vi "matlab_create.vi"(4 "error in":errorcluster, 5 "creator":string="h5labview", 6 "platform":string="LabVIEW", 7 "path in":path) -> (0 "error out":errorcluster, 3 "path out":path)   [LabVIEW 2019]
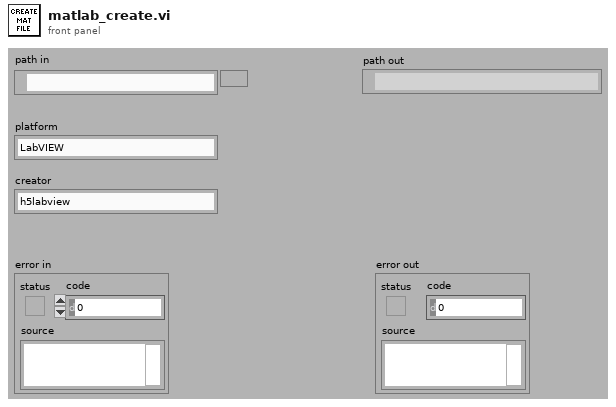
[diagram p1: front panel]
types:
  T1 = enum16{"big-endian, network order", "native, host order", "little-endian"}
  T2 = enum16{"open", "replace", "create", "open or create", "replace or create", "replace or create with confirmation"}
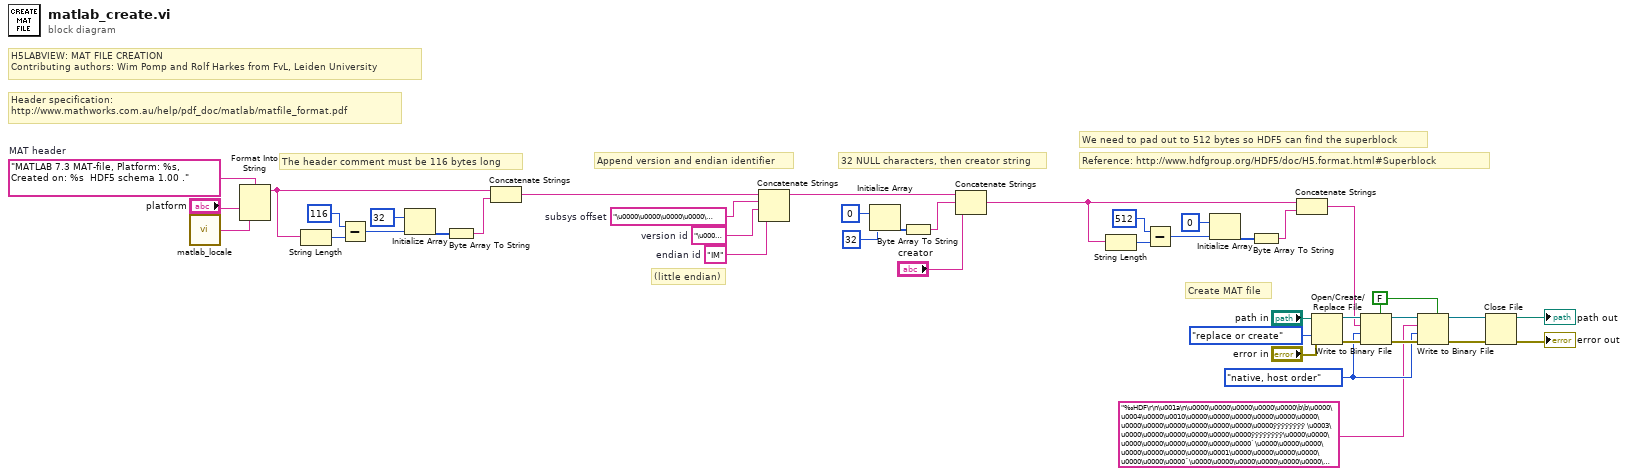
[diagram p0: block diagram]
diagram:
  w4 = T1."native, host order" ("byte order (0:big-endian, network order)")
  w9 = FALSE ("prepend array or string size? (T)")
  w26 = "IM"  # endian id
  w25 = "\u0000\u0002"  # version id
  w27 = "\u0000\u0000\u0000\u0000\u0000\u0000\u0000\u0000"  # subsys offset
  w42 = "MATLAB 7.3 MAT-file, Platform: %s, Created on: %s  HDF5 schema 1.00 ."  # MAT header
  # "H5LABVIEW: MAT FILE CREATION \nContributing authors: Wim Pomp and Rolf Harkes from FvL, Leiden University"
  # "Create MAT file"
  # "Header specification:\nhttp://www.mathworks.com.au/help/pdf_doc/matlab/matfile_format.pdf"
  # "32 NULL characters, then creator string"
  # "(little endian)"
  # "Append version and endian identifier"
  # "The header comment must be 116 bytes long"
  # "We need to pad out to 512 bytes so HDF5 can find the superblock"
  # "Reference: http://www.hdfgroup.org/HDF5/doc/H5.format.html#Superblock"
  n1 = call "matlab_locale.vi"() -> ("datetime"=w16:string)
  n2 = Format Into String(format string=w42, "platform", w16) -> (resulting string=w36:string)  [unwired: 2 in, 1 out]
  n3 = String Length(string=w36) -> (length=w41:i32)
  n4 = Subtract(x=116 ("length"), y=w41) -> (x-y=w39:i32)
  n5 = Initialize Array(u8 32 ("length"), w39) -> (w38:u8[])
  n6 = Byte Array To String(unsigned byte array=w38) -> (string=w35:string)
  n7 = Concatenate Strings(w36, w35) -> (w28:string)
  n8 = Concatenate Strings(w28, w27, w25, w26) -> (w21:string)
  n9 = Initialize Array(u8 0 ("length"), 32 ("dimension size")) -> (w24:u8[])
  n10 = Byte Array To String(unsigned byte array=w24) -> (string=w20:string)
  n11 = Concatenate Strings(w21, w20, "creator") -> (w19:string)
  n12 = String Length(string=w19) -> (length=w30:i32)
  n13 = Subtract(x=512 ("length"), y=w30) -> (x-y=w32:i32)
  n14 = Initialize Array(u8 0 ("length"), w32) -> (w33:u8[])
  n15 = Byte Array To String(unsigned byte array=w33) -> (string=w29:string)
  n16 = Concatenate Strings(w19, w29) -> (w12:string)
  n17 = Open/Create/Replace File(file path (use dialog)="path in", error in="error in", operation (0:open)=T2."replace or create") -> (refnum out=w13:refnum<file>, error out=w11:errorcluster)  [unwired: 3 in, 1 out]
  n18 = Write to Binary File(file (use dialog)=w13, data=w12, error in=w11, 5:w9, 9:w4) -> (refnum out=w8:refnum<file>, error out=w7:errorcluster)  [unwired: 1 in, 1 out]
  n19 = Write to Binary File(file (use dialog)=w8, data="‰HDF\r\n\u001a\n\u0000\u0000\u0000\u0000\u0000\b\b\u0000\u0004\u0000\u0010\u0000\u0000\u0000\u0000\u0000\u0000\u0000\u0000\u0000\u0000\u0000\u0000\u0000ÿÿÿÿÿÿÿÿ \u0003\u0000\u0000\u0000\u0000\u0000\u0000ÿÿÿÿÿÿÿÿ\u0000\u0000\u0000\u0000\u0000\u0000\u0000\u0000`\u0000\u0000\u0000\u0000\u0000\u0000\u0000\u0001\u0000\u0000\u0000\u0000\u0000\u0000\u0000ˆ\u0000\u0000\u0000\u0000\u0000\u0000\u0000¨\u0002\u0000\u0000\u0000\u0000\u0000\u0000\u0001\u0000\u0001\u0000\u0001\u0000\u0000\u0000\u0018\u0000\u0000\u0000\u0000\u0000\u0000\u0000\u0011\u0000\u0010\u0000\u0000\u0000\u0000\u0000ˆ\u0000\u0000\u0000\u0000\u0000\u0000\u0000¨\u0002\u0000\u0000\u0000\u0000\u0000\u0000TREE\u0000\u0000\u0000\u0000ÿÿÿÿÿÿÿÿÿÿÿÿÿÿÿÿ\u0000\u0000\u0000\u0000\u0000\u0000\u0000\u0000\u0000\u0000\u0000\u0000\u0000\u0000\u0000\u0000\u0000\u0000\u0000\u0000\u0000\u0000\u0000\u0000\u0000\u0000\u0000\u0000\u0000\u0000\u0000\u0000\u0000\u0000\u0000\u0000\u0000\u0000\u0000\u0000\u0000\u0000\u0000\u0000\u0000\u0000\u0000\u0000\u0000\u0000\u0000\u0000\u0000\u0000\u0000\u0000\u0000\u0000\u0000\u0000\u0000\u0000\u0000\u0000\u0000\u0000\u0000\u0000\u0000\u0000\u0000\u0000\u0000\u0000\u0000\u0000\u0000\u0000\u0000\u0000\u0000\u0000\u0000\u0000\u0000\u0000\u0000\u0000\u0000\u0000\u0000\u0000\u0000\u0000\u0000\u0000\u0000\u0000\u0000\u0000\u0000\u0000\u0000\u0000\u0000\u0000\u0000\u0000\u0000\u0000\u0000\u0000\u0000\u0000\u0000\u0000\u0000\u0000\u0000\u0000\u0000\u0000\u0000\u0000\u0000\u0000\u0000\u0000\u0000\u0000\u0000\u0000\u0000\u0000\u0000\u0000\u0000\u0000\u0000\u0000\u0000\u0000\u0000\u0000\u0000\u0000\u0000\u0000\u0000\u0000\u0000\u0000\u0000\u0000\u0000\u0000\u0000\u0000\u0000\u0000\u0000\u0000\u0000\u0000\u0000\u0000\u0000\u0000\u0000\u0000\u0000\u0000\u0000\u0000\u0000\u0000\u0000\u0000\u0000\u0000\u0000\u0000\u0000\u0000\u0000\u0000\u0000\u0000\u0000\u0000\u0000\u0000\u0000\u0000\u0000\u0000\u0000\u0000\u0000\u0000\u0000\u0000\u0000\u0000\u0000\u0000\u0000\u0000\u0000\u0000\u0000\u0000\u0000\u0000\u0000\u0000\u0000\u0000\u0000\u0000\u0000\u0000\u0000\u0000\u0000\u0000\u0000\u0000\u0000\u0000\u0000\u0000\u0000\u0000\u0000\u0000\u0000\u0000\u0000\u0000\u0000\u0000\u0000\u0000\u0000\u0000\u0000\u0000\u0000\u0000\u0000\u0000\u0000\u0000\u0000\u0000\u0000\u0000\u0000\u0000\u0000\u0000\u0000\u0000\u0000\u0000\u0000\u0000\u0000\u0000\u0000\u0000\u0000\u0000\u0000\u0000\u0000\u0000\u0000\u0000\u0000\u0000\u0000\u0000\u0000\u0000\u0000\u0000\u0000\u0000\u0000\u0000\u0000\u0000\u0000\u0000\u0000\u0000\u0000\u0000\u0000\u0000\u0000\u0000\u0000\u0000\u0000\u0000\u0000\u0000\u0000\u0000\u0000\u0000\u0000\u0000\u0000\u0000\u0000\u0000\u0000\u0000\u0000\u0000\u0000\u0000\u0000\u0000\u0000\u0000\u0000\u0000\u0000\u0000\u0000\u0000\u0000\u0000\u0000\u0000\u0000\u0000\u0000\u0000\u0000\u0000\u0000\u0000\u0000\u0000\u0000\u0000\u0000\u0000\u0000\u0000\u0000\u0000\u0000\u0000\u0000\u0000\u0000\u0000\u0000\u0000\u0000\u0000\u0000\u0000\u0000\u0000\u0000\u0000\u0000\u0000\u0000\u0000\u0000\u0000\u0000\u0000\u0000\u0000\u0000\u0000\u0000\u0000\u0000\u0000\u0000\u0000\u0000\u0000\u0000\u0000\u0000\u0000\u0000\u0000\u0000\u0000\u0000\u0000\u0000\u0000\u0000\u0000\u0000\u0000\u0000\u0000\u0000\u0000\u0000\u0000\u0000\u0000\u0000\u0000\u0000\u0000\u0000\u0000\u0000\u0000\u0000\u0000\u0000\u0000\u0000\u0000\u0000\u0000\u0000\u0000\u0000\u0000\u0000\u0000..." ("data 2"), error in=w7, 5:w9, 9:w4) -> (refnum out=w5:refnum<file>, error out=w6:errorcluster)  [unwired: 1 in, 1 out]
  n20 = Close File(refnum=w5, error in=w6) -> (path=→"path out":path, error out=→"error out":errorcluster)
